vi "ProyectoControlDeNivel_conAlarmaSonora - Cristhian Tipan.vi"() -> ()   [LabVIEW 2020]
panel:
  in  "?":bool
  out "x < y?":bool
  out "x > y?":bool
  in  "y 2":dbl
  in  "y":dbl
  out "Waveform Chart":dbl(graph)
  out "Tank":dbl(slide) scale=0.0..100.0
  in  "Dial":dbl(knob) scale=0.0..100.0
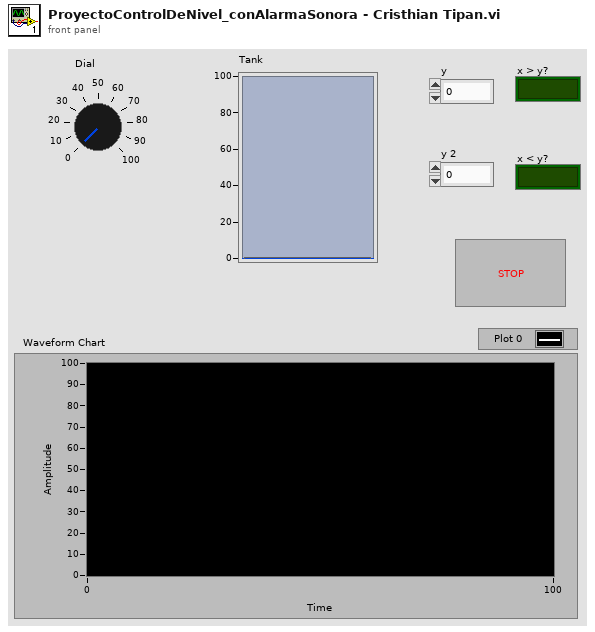
[diagram p1: front panel]
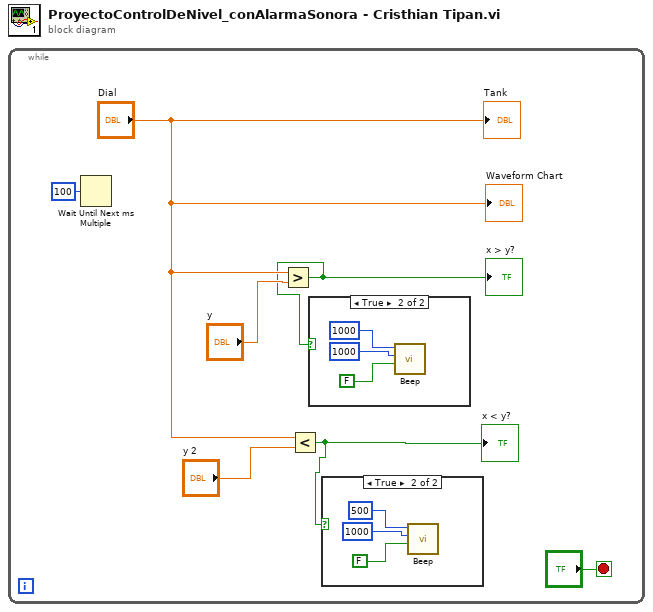
[diagram p0: block diagram]
diagram:
  n1 = while {
    stop <- "?" stop-if-true
    n2 = Wait Until Next ms Multiple(millisecond multiple=100) -> ()  [unwired: 1 out]
    n3 = Greater?(x="Dial", y="y") -> (0:w2:bool)
    "x > y?" <- w2
    n4 = Less?(x="Dial", y="y 2") -> (x < y?=w1:bool)
    "x < y?" <- w1
    n5 = case shown="True" w2 {
      frame False {
      }
      frame True {
        n6 = call <vilib>:"Beep.vi"("use system alert? (T)"=FALSE, "duration (msec)"=u32 1000 ("frequency (Hz)"), "frequency (Hz)"=u32 1000) -> ()  [unwired: 9 in]
      }
    }
    n7 = case shown="True" w1 {
      frame False {
      }
      frame True {
        n8 = call <vilib>:"Beep.vi"("use system alert? (T)"=FALSE, "duration (msec)"=u32 1000 ("frequency (Hz)"), "frequency (Hz)"=u32 500) -> ()  [unwired: 9 in]
      }
    }
    "Tank" <- "Dial"
    "Waveform Chart" <- "Dial"
  }
